vi "Main.vi"() -> ()   [LabVIEW 2020, in "helloWServer.lvlib" / "helloWServer.lvclass"]
uses:
  helloWServer.lvclass
  typeDefs/Server State Data.ctl
  helloWServer.lvclass/helloWServer.ctl
panel:
  in  "Stop":bool
  in  "Server Address":string="0.0.0.0:50051"
  in  "Server Certificate File (.crt)":path
  in  "Server Key File (.key)":path
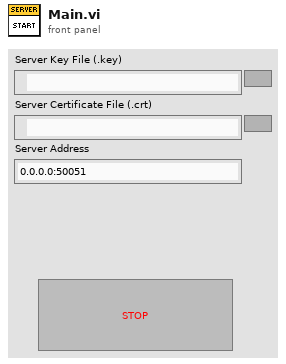
[diagram p1: front panel]
types:
  T1 = typedef "helloWServer.lvlib/helloWServer.lvclass/Server State Data.ctl" = cluster{"Data":string}
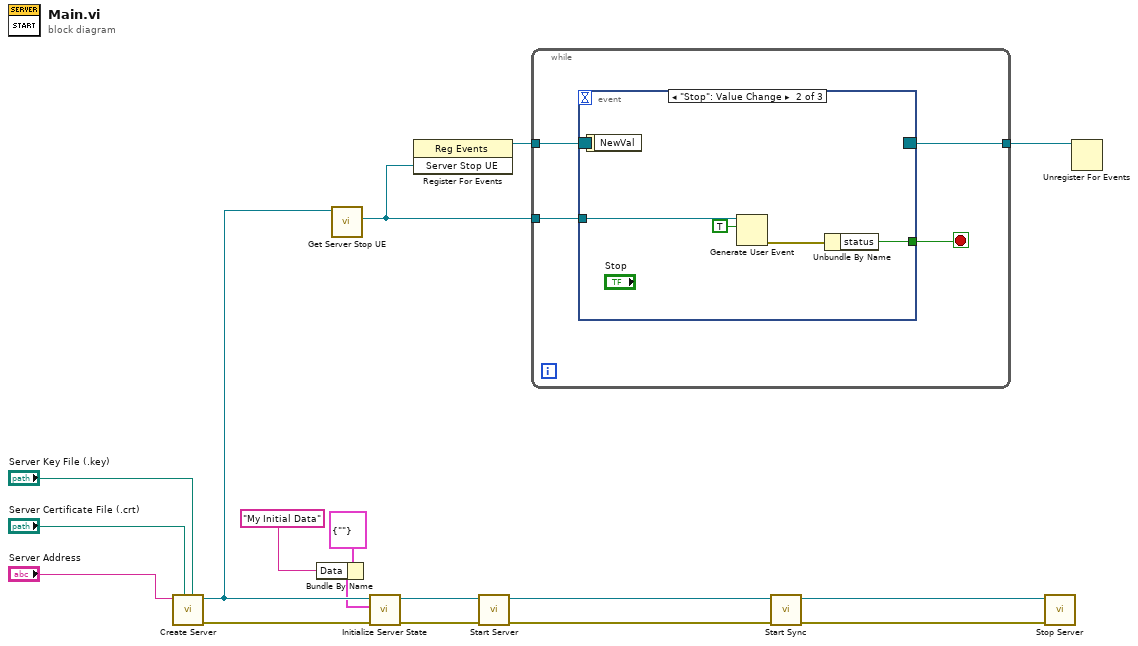
[diagram p0: block diagram]
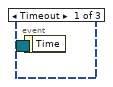
[diagram p2: hidden frame]
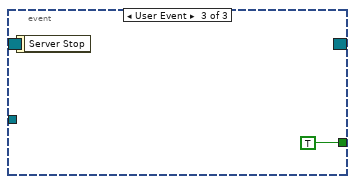
[diagram p3: hidden frame]
diagram:
  n1 = call "Create Server.vi"("Server Key File (.key)"="Server Key File (.key)", "Server Certificate File (.crt)"="Server Certificate File (.crt)", "Server Address"="Server Address") -> ("error out"=w7:errorcluster, "gRPC Server out"=w4:refnum<class "helloWServer.lvclass">)  [unwired: 7 in]
  n2 = Bundle By Name(cluster=T1 {"Data"=""} ("Initial State"), "Data"="My Initial Data") -> (w2:T1)
  n3 = call "Get Server Stop UE.vi"("OOP Server in"=w4) -> ("Server Stop UE"=w8:refnum<user-event>)  [unwired: 9 in, 1 out]
  n4 = call "Initialize Server State.vi"("error in (no error)"=w7, "Initial State"=w2, "gRPC Server in"=w4) -> ("error out"=w6:errorcluster, "gRPC Server out"=w5:refnum<class "helloWServer.lvclass">)  [unwired: 7 in]
  n5 = register-events(w8) -> (reference out=w10:refnum<event-registration>)  [unwired: 2 in, 1 out]
  n6 = call "Start Server.vi"("error in (no error)"=w6, "gRPC Server in"=w5) -> ("error out"=w17:errorcluster, "gRPC Server out"=w16:refnum<class "helloWServer.lvclass">)  [unwired: 8 in]
  n7 = while {
    tunnel: w8 -> [w21]
    tunnel: w10 -> [w20]
    tunnel: [w18] -> w9
    stop <- w19 stop-if-true
    n8 = event shown="[1] \"Stop\": Value Change" {
      selector: w20 -> [_ _ _]
      dyn-events: [_ _ _] -> w18
      timeout: _ -> [_ _ _]
      tunnel: w21 -> [_ w25 _]
      tunnel: [_ w22 TRUE] -> w19
      event Timeout {
        n9 = event-data() -> ()  [unwired: 1 in, 1 out]
      }
      event "Stop": Value Change {
        n10 = event-data() -> ()  [unwired: 1 in, 1 out]
        n11 = Generate User Event(user event=w25, event data cluster=TRUE ("event data")) -> (error out=w23:errorcluster)  [unwired: 2 in, 1 out]
        n12 = Unbundle By Name(w23) -> ("status"=w22:bool)
      }
      event User Event {
        n13 = event-data() -> ()  [unwired: 1 in, 1 out]
      }
    }
  }
  n14 = call "Start Sync.vi"("error in (no error)"=w17, "gRPC Server in"=w16) -> ("error out"=w15:errorcluster, "gRPC Server out"=w14:refnum<class "helloWServer.lvclass">)  [unwired: 8 in]
  n15 = call "Stop Server.vi"("error in (no error)"=w15, "gRPC Server in"=w14) -> ()  [unwired: 9 in, 1 out]
  n16 = Unregister For Events(event registration refnum=w9) -> ()  [unwired: 1 in, 1 out]
